vi "Teleop.vi"(10 "Match Info":T7={"Autonomous Elapsed Seconds"=0.0, "TeleOp Elapsed Seconds"=0.0, "Disabled Elapsed Seconds"=0.0, "Visited Autonomous"=FALSE, "Visited TeleOp"=FALSE, "Visited Disabled"=FALSE, "Autonomous Settings"={"Autonomous Style"=enum."Independent", "VI Refnum"=refnum}}, 11 "Call Context":T8) -> ()   [LabVIEW 2013]
doc: "This VI is called for each TeleOp packet received from the DS where the robot is not disabled. It is often used to read from the joysticks and update I/O or to update setpoints for timed control loops. It should complete and return within 20 milliseconds or it may miss DS packets."
uses:
  <vilib>/Rock Robotics/WPI/DriverStation/WPI_DriverStationDerivedRobotMode.ctl
  <vilib>/Rock Robotics/WPI/DriverStation/WPI_DriverStationMatch Info.ctl
  <vilib>/Rock Robotics/WPI/Joystick/WPI_JoystickButtonState.ctl
  <vilib>/Rock Robotics/WPI/Relay/WPI_RelayDevRef.ctl
  <vilib>/Rock Robotics/SystemInterfaces/DIO/FPGA_DIORelayChannel.ctl
  <vilib>/Rock Robotics/SystemInterfaces/Typedef/FPGA_TypedefDigitalModule.ctl
  <vilib>/Rock Robotics/WPI/Relay/WPI_RelayDirection.ctl
  <vilib>/Rock Robotics/WPI/DriverStation/DriverStationLCD/WPI_DriverStationLCDLCDLine.ctl
  <vilib>/Rock Robotics/WPI/Relay/WPI_RelayValue.ctl
  Robot Global Data.vi
  <vilib>/addons/control/pid/pid.llb/PID (DBL).vi
  <vilib>/Rock Robotics/WPI/RobotDrive/WPI_RobotDriveArcadeDrive_Standard(NoSaturation).vi
  <vilib>/Rock Robotics/WPI/RobotDrive/WPI_RobotDriveGetSetRefNum.vi
  <vilib>/Rock Robotics/WPI/Joystick/WPI_JoystickGetSetRefNum.vi
  <vilib>/addons/control/pid/NI_PID_pid.lvlib
panel:
  out "trimmert_watch":i32
  in  "steering_trim":dbl(slide) scale=1.0..-1.0
  in  "Ball_Sucker_Reducer":dbl=0.8
  in  "shooter_speed_med_high":dbl(slide)=0.6 scale=0.0..1.0
  in  "shooter_speed_med_low":dbl(slide)=0.35 scale=0.0..1.0
  in  "shooter_speed_high":dbl(slide)=1.0 scale=0.0..1.0
  in  "shooter_speed_low":dbl(slide)=0.25 scale=0.0..1.0
  in  "Camera_Tilt_Position":dbl(slide)=0.55 scale=1.0..-1.0
  in  "Shoot_Feeder_Reducer":dbl=0.9
  out "Battery_Relay":T1={"DevStatus"={"status"=FALSE, "code"=0, "source"=""}, "Relay Channel"=enum."Invalid", "Digital Module"=enum."Digital Module 1", "Relay Direction"=enum."Both directions"}
  in  "Camera_Pan_Position":dbl(slide)=-1.0 scale=1.0..-1.0
  in  "ARM_HOME":dbl(slide)=0.53 scale=1.0..-1.0
  in  "ARM_REV_LIMIT":dbl(slide)=-0.2 scale=1.0..-1.0
  in  "Drive_Y_Speed":dbl
  in  "Drive_X_Speed":dbl=1.5
  in  "Feeder_Arm_Speed":dbl
  in  "Sucker_Speed":dbl
  in  "Shooter_Speed":dbl=1.5
  in  "Shoot_Feeder_Speed":dbl=1.5
  in  "Ball_Sucker_Threshold":i64=10
  in  "Ball_Sucker_Delay_ms":i64=100
  in  "Ball_Sucker_Counter":i64
  in  "Steering_Reduce":dbl=2.0
  in  "Shooter_Angle_Raw":dbl
  in  "Camera_SIDE_Val":dbl=0.5
  in  "Camera_FWD_Val":dbl
  in  "ARM_FWD_LIMIT":dbl(slide)=0.53 scale=1.0..-1.0
  in  "Drive_Reduce":dbl=0.75
  out "JS1_BTNS":T5
  out "JS1_AXES":T6
  out "JS2_BTNS":T5
  out "JS2_AXES":T6
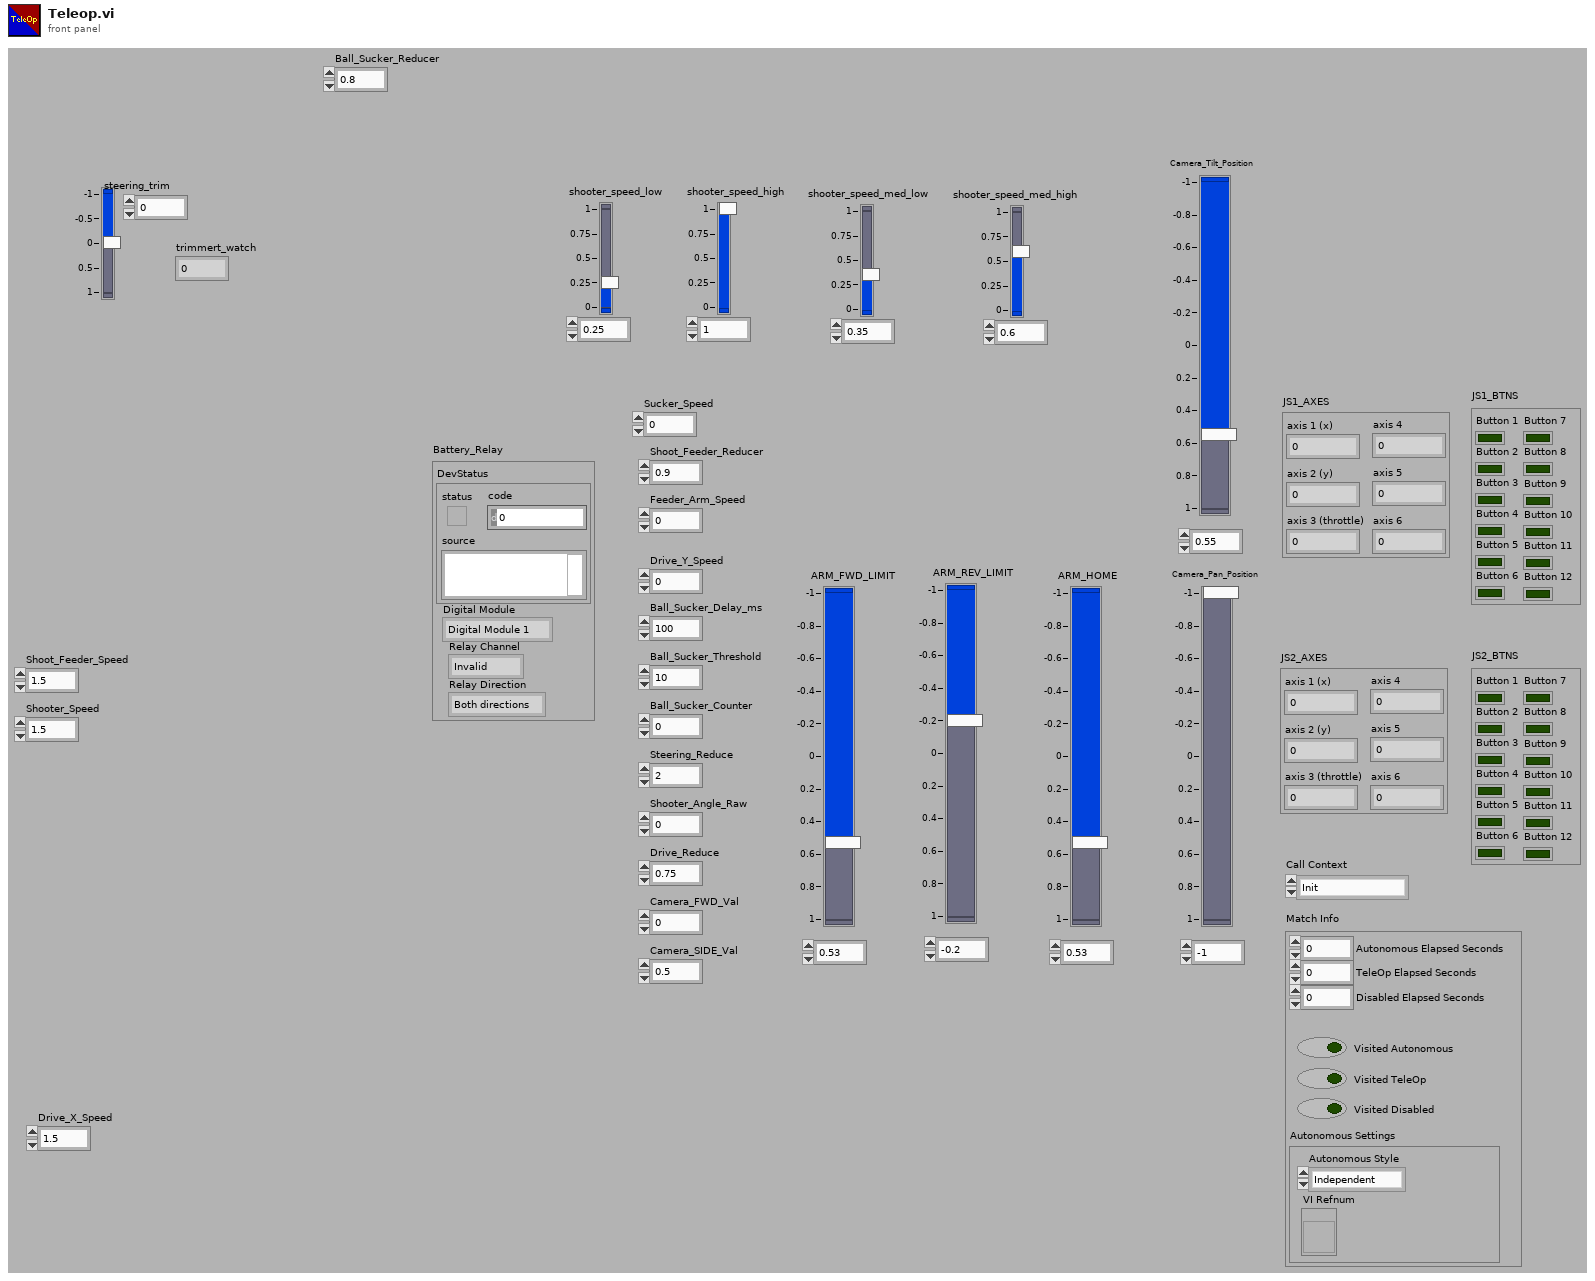
[diagram p1: front panel]
types:
  T1 = typedef "WPI_RelayDevRef.ctl" = cluster{"DevStatus":errorcluster, "Relay Channel":T2, "Digital Module":T3, "Relay Direction":T4}
  T2 = typedef "FPGA_DIORelayChannel.ctl" = enum8{"Relay 1", "Relay 2", "Relay 3", "Relay 4", "Relay 5", "Relay 6", "Relay 7", "Relay 8", "Invalid"}
  T3 = typedef "FPGA_TypedefDigitalModule.ctl" = enum16{"Digital Module 1", "Digital Module 2"}
  T4 = typedef "WPI_RelayDirection.ctl" = enum16{"Both directions", "Forward only", "Reverse only"}
  T5 = typedef "WPI_JoystickButtonState.ctl" = cluster{"Button 1":bool, "Button 2":bool, "Button 3":bool, "Button 4":bool, "Button 5":bool, "Button 6":bool, "Button 7":bool, "Button 8":bool, "Button 9":bool, "Button 10":bool, "Button 11":bool, "Button 12":bool}
  T6 = cluster{"axis 1 (x)":dbl, "axis 2 (y)":dbl, "axis 3 (throttle)":dbl, "axis 4":dbl, "axis 5":dbl, "axis 6":dbl}
  T7 = typedef "WPI_DriverStationMatch Info.ctl" = cluster{"Autonomous Elapsed Seconds":dbl, "TeleOp Elapsed Seconds":dbl, "Disabled Elapsed Seconds":dbl, "Visited Autonomous":bool, "Visited TeleOp":bool, "Visited Disabled":bool, "Autonomous Settings":cluster{"Autonomous Style":enum16{"Iterative", "Independent"}, "VI Refnum":refnum<vi>}}
  T8 = typedef "WPI_DriverStationDerivedRobotMode.ctl" = enum16{"Init", "Execute", "Stop"}
  T9 = typedef "WPI_DriverStationLCDLCDLine.ctl" = enum16{"Main - Line 1", "User - Line 2", "User - Line 3", "User - Line 4", "User - Line 5", "User - Line 6"}
  T10 = typedef "WPI_JoystickDevRef.ctl" = cluster{"Device":T11}
  T11 = typedef "WPI_JoystickDeviceEnum.ctl" = enum16{"USB 1", "USB 2", "USB 3", "USB 4", "Kinect 1", "Kinect 2"}
  T12 = typedef "WPI_MotorControlDeviceRef.ctl" = cluster{"DeviceStatus":errorcluster, "Type":enum16{"PWM", "CAN"}, "PWM":cluster{"Digital Module":T3, "PWM Channel":T13, "DeadBand":T14}, "CAN":cluster{"Device Number":u8, "Control Mode":T15, "Semaphore":T16, "Max Vout":dbl}, "Invert":bool, "TransformRef":T17, "InvTransformRef":T17}
  T13 = typedef "FPGA_DIOPWMChannel.ctl" = enum8{"PWM 1", "PWM 2", "PWM 3", "PWM 4", "PWM 5", "PWM 6", "PWM 7", "PWM 8", "PWM 9", "PWM 10", "Invalid"}
  T14 = typedef "WPI_PWMDeadband.ctl" = cluster{"Name":string, "maxPositivePwm":i32, "minPositivePwm":i32, "centerPwm":i32, "maxNegativePwm":i32, "minNegativePwm":i32, "angularRange":u16}
  T15 = typedef "WPI_CANJaguar_ControlMode.ctl" = enum8{"Percent VBus", "Current", "Speed", "Position", "Voltage"}
  T16 = typedef "Semaphore RefNum" = refnum<k1>
  T17 = typedef "WPI_PWMTransform_ConPane.ctl" = refnum<vi>
  T18 = typedef "WPI_RobotDriveDevRef.ctl" = cluster{"DevStatus":errorcluster, "Motors[]":T12[], "Square Inputs":bool, "Max Output":dbl, "Isochronous":bool}
  T19 = cluster{"proportional gain (Kc)":dbl, "integral time (Ti, min)":dbl, "derivative time (Td, min)":dbl}
  T20 = typedef "WPI_AnalogChannelDevRef.ctl" = cluster{"DevStatus":errorcluster, "Analog Module":T21, "Analog Channel":T22}
  T21 = typedef "FPGA_TypedefAnalogModule.ctl" = enum16{"Analog Module 1", "Analog Module 2"}
  T22 = typedef "FPGA_AIChannel.ctl" = enum8{"AI 1", "AI 2", "AI 3", "AI 4", "AI 5", "AI 6", "AI 7", "AI 8", "Invalid"}
  T23 = typedef "WPI_RelayValue.ctl" = enum16{"Off", "On", "Forward", "Reverse"}
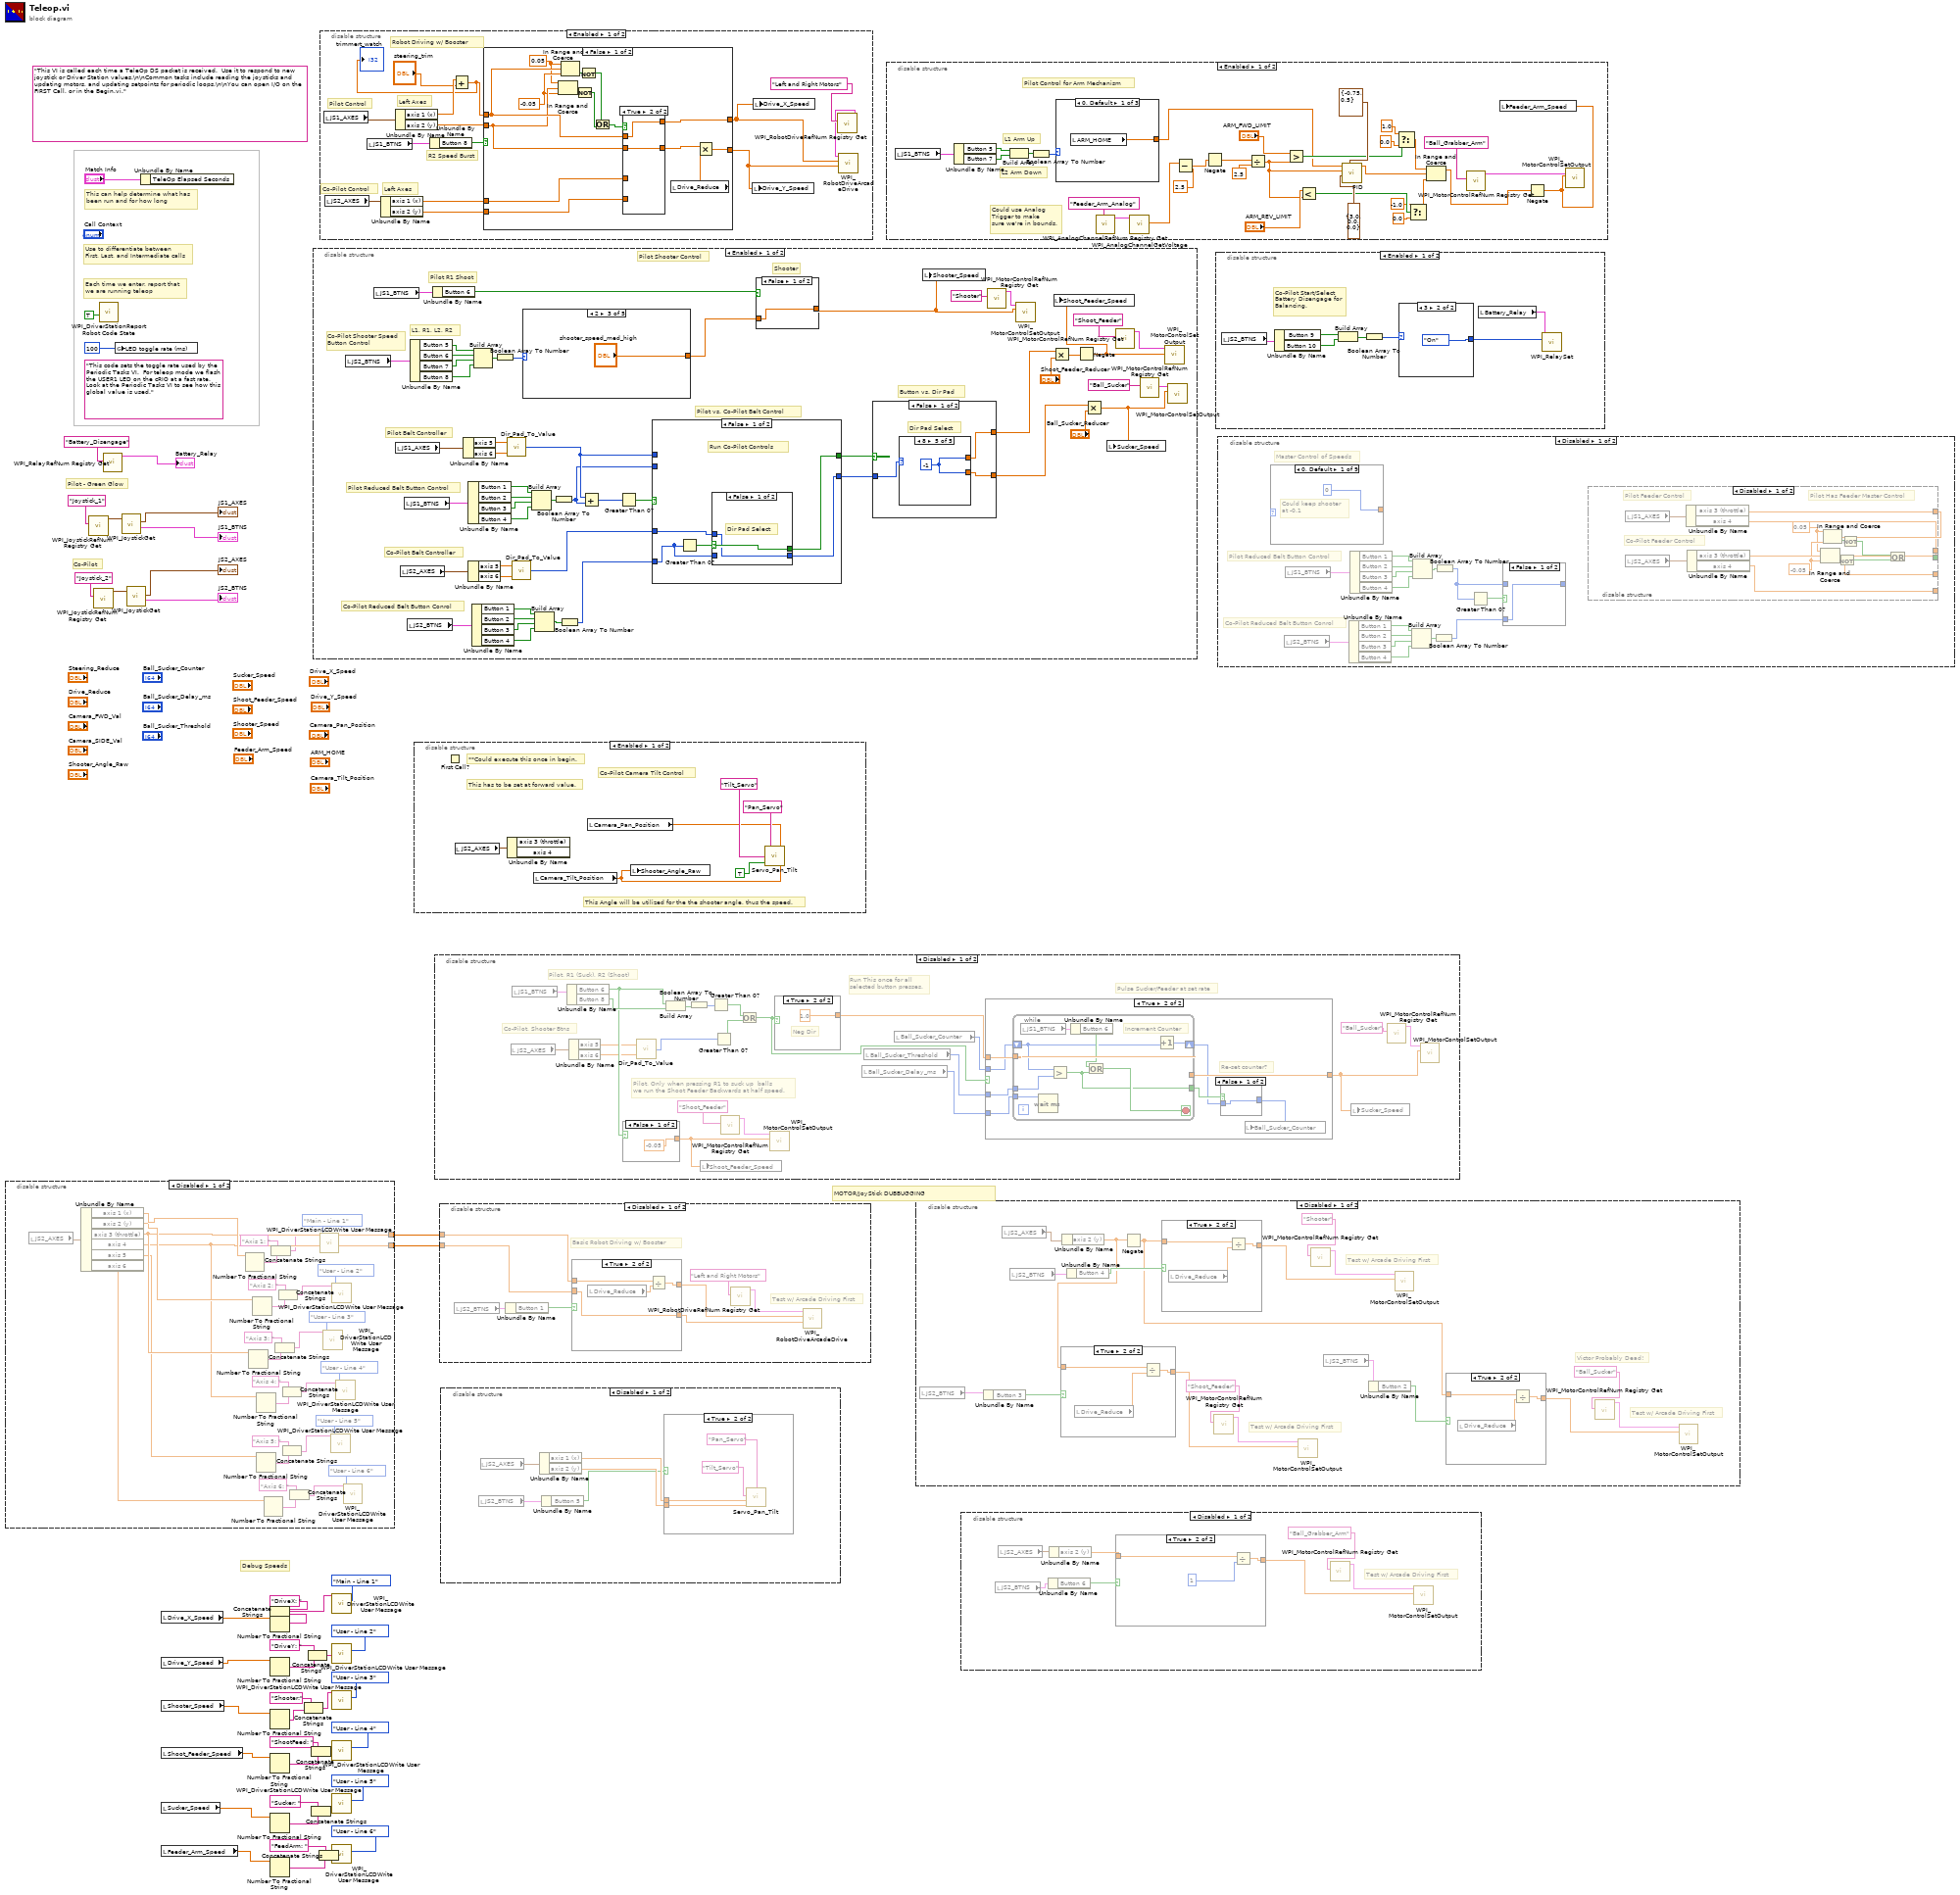
[diagram p0: block diagram]
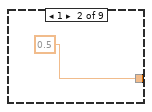
[diagram p4: hidden frame]
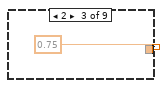
[diagram p5: hidden frame]
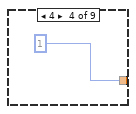
[diagram p6: hidden frame]
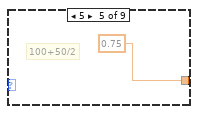
[diagram p7: hidden frame]
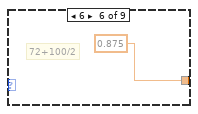
[diagram p8: hidden frame]
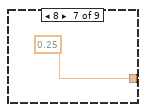
[diagram p9: hidden frame]
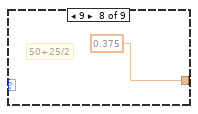
[diagram p10: hidden frame]
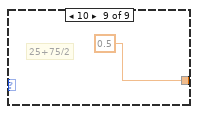
[diagram p11: hidden frame]
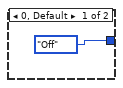
[diagram p13: hidden frame]
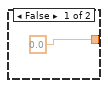
[diagram p16: hidden frame]
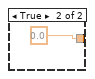
[diagram p18: hidden frame]
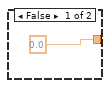
[diagram p19: hidden frame]
diagram:
  (unwired) "This code sets the toggle rate used by the Periodic Tasks VI.  For teleop mode we flash the USER1 LED on the cRIO at a fast rate.  Look at the Periodic Tasks VI to see how this global value is used."
  (unwired) "This VI is called each time a TeleOp DS packet is received.  Use it to respond to new joystick or Driver Station values.\n\nCommon tasks include reading the joysticks and updating motors, and updating setpoints for periodic loops.\n\nYou can open I/O on the FIRST Call, or in the Begin.vi."
  # "Debug Speeds"
  # "Co-Pilot"
  # "Pilot - Green Glow"
  # "MOTOR/JoyStick DUBBUGGING"
  # "Each time we enter, report that\nwe are running teleop"
  # "Use to differentiate between\nFirst, Last, and Intermediate calls"
  # "This can help determine what has\nbeen run and for how long"
  n1 = disable-structure shown="Disabled" {
    disable-tunnel: [w73 _] -> w34
    disable-tunnel: [w72 _] -> w33
    frame Disabled {
      n2 = local read "JS2_AXES"() -> (w76:T6)
      n3 = Unbundle By Name(w76) -> ("axis 1 (x)"=w75:dbl, "axis 2 (y)"=w74:dbl, "axis 3 (throttle)"=w73:dbl, "axis 4"=w72:dbl, "axis 5"=w71:dbl, "axis 6"=w70:dbl)
      n4 = Number To Fractional String(number=w75) -> (F-format string=w67:string)  [unwired: 3 in]
      n5 = Number To Fractional String(number=w73) -> (F-format string=w59:string)  [unwired: 3 in]
      n6 = Number To Fractional String(number=w74) -> (F-format string=w65:string)  [unwired: 3 in]
      n7 = Number To Fractional String(number=w72) -> (F-format string=w57:string)  [unwired: 3 in]
      n8 = Number To Fractional String(number=w71) -> (F-format string=w51:string)  [unwired: 3 in]
      n9 = Number To Fractional String(number=w70) -> (F-format string=w49:string)  [unwired: 3 in]
      n10 = Concatenate Strings("Axis 1: ", w67) -> (w64:string)
      n11 = Concatenate Strings("Axis 3: ", w59) -> (w56:string)
      n12 = Concatenate Strings("Axis 2: ", w65) -> (w62:string)
      n13 = Concatenate Strings("Axis 4: ", w57) -> (w54:string)
      n14 = Concatenate Strings("Axis 5: ", w51) -> (w48:string)
      n15 = Concatenate Strings("Axis 6: ", w49) -> (w46:string)
      n16 = call <vilib>:"WPI_DriverStationLCDWrite User Message.vi"("line text"=w64, "line"=WPI_DriverStationLCDLCDLine."Main - Line 1") -> ()  [unwired: 13 in, 1 out]
      n17 = call <vilib>:"WPI_DriverStationLCDWrite User Message.vi"("line text"=w56, "line"=WPI_DriverStationLCDLCDLine."User - Line 3") -> ()  [unwired: 13 in, 1 out]
      n18 = call <vilib>:"WPI_DriverStationLCDWrite User Message.vi"("line text"=w48, "line"=WPI_DriverStationLCDLCDLine."User - Line 5") -> ()  [unwired: 13 in, 1 out]
      n19 = call <vilib>:"WPI_DriverStationLCDWrite User Message.vi"("line text"=w62, "line"=WPI_DriverStationLCDLCDLine."User - Line 2") -> ()  [unwired: 13 in, 1 out]
      n20 = call <vilib>:"WPI_DriverStationLCDWrite User Message.vi"("line text"=w54, "line"=WPI_DriverStationLCDLCDLine."User - Line 4") -> ()  [unwired: 13 in, 1 out]
      n21 = call <vilib>:"WPI_DriverStationLCDWrite User Message.vi"("line text"=w46, "line"=WPI_DriverStationLCDLCDLine."User - Line 6") -> ()  [unwired: 13 in, 1 out]
    }
    frame Enabled {
    }
  }
  n22 = call <vilib>:"WPI_JoystickRefNum Registry Get.vi"("refnum name"="Joystick_1") -> ("JoystickDevRef"=w38:T10)  [unwired: 1 in, 9 out]
  n23 = call <vilib>:"WPI_JoystickRefNum Registry Get.vi"("refnum name"="Joystick_2") -> ("JoystickDevRef"=w40:T10)  [unwired: 1 in, 9 out]
  n24 = call <vilib>:"WPI_DriverStationReport Robot Code State.vi"("TeleOp"=TRUE ("Autonomous")) -> ()  [unwired: 10 in, 1 out]
  n25 = call <vilib>:"WPI_RelayRefNum Registry Get.vi"("refnum name"="Battery_Disengage") -> ("RelayDevRef"=→"Battery_Relay":T1)  [unwired: 9 in, 1 out]
  n26 = global write "Robot Global Data.vi" "LED toggle rate (ms)"(u32 100 ("LED ms toggle rate")) -> ()
  n27 = call <vilib>:"WPI_JoystickGet.vi"("JoystickDevRef"=w38) -> ("Buttons"=→"JS1_BTNS":T5, "Axes"=→"JS1_AXES":T6)  [unwired: 1 in, 4 out]
  n28 = call <vilib>:"WPI_JoystickGet.vi"("JoystickDevRef"=w40) -> ("Buttons"=→"JS2_BTNS":T5, "Axes"=→"JS2_AXES":T6)  [unwired: 1 in, 4 out]
  n29 = Unbundle By Name("Match Info") -> ()  [unwired: 1 out]
  n30 = local read "Drive_X_Speed"() -> (w9:dbl)
  n31 = local read "Drive_Y_Speed"() -> (w8:dbl)
  n32 = local read "Shooter_Speed"() -> (w7:dbl)
  n33 = local read "Shoot_Feeder_Speed"() -> (w6:dbl)
  n34 = local read "Sucker_Speed"() -> (w5:dbl)
  n35 = local read "Feeder_Arm_Speed"() -> (w4:dbl)
  n36 = Number To Fractional String(number=w9) -> (F-format string=w30:string)  [unwired: 3 in]
  n37 = Concatenate Strings("DriveX: ", w30) -> (w27:string)
  n38 = Number To Fractional String(number=w8) -> (F-format string=w28:string)  [unwired: 3 in]
  n39 = Number To Fractional String(number=w7) -> (F-format string=w3:string)  [unwired: 3 in]
  n40 = Number To Fractional String(number=w6) -> (F-format string=w21:string)  [unwired: 3 in]
  n41 = Number To Fractional String(number=w5) -> (F-format string=w15:string)  [unwired: 3 in]
  n42 = Number To Fractional String(number=w4) -> (F-format string=w13:string)  [unwired: 3 in]
  n43 = Concatenate Strings("Shooter:", w3) -> (w20:string)
  n44 = Concatenate Strings("DriveY: ", w28) -> (w25:string)
  n45 = Concatenate Strings("ShootFeed: ", w21) -> (w18:string)
  n46 = Concatenate Strings("Sucker: ", w15) -> (w12:string)
  n47 = disable-structure shown="Enabled" {
    frame Enabled {
      # "Button vs. Dir Pad"
      # "Pilot vs. Co-Pilot Belt Control"
      # "Co-Pilot Belt Controller"
      # "L1, R1, L2, R2"
      # "Co-Pilot Reduced Belt Button Conrol"
      # "Pilot Reduced Belt Button Control"
      # "Pilot Belt Controller"
      # "Co-Pilot Shooter Speed\nButton Control"
      # "Pilot R1 Shoot"
      # "Shooter"
      # "Pilot Shooter Control"
      n48 = local read "JS2_BTNS"() -> (w108:T5)
      n49 = local read "JS1_BTNS"() -> (w126:T5)
      n50 = local read "JS1_AXES"() -> (w105:T6)
      n51 = local read "JS2_AXES"() -> (w90:T6)
      n52 = local read "JS1_BTNS"() -> (w104:T5)
      n53 = local read "JS2_BTNS"() -> (w93:T5)
      n54 = Unbundle By Name(w108) -> ("Button 5"=w114:bool, "Button 6"=w113:bool, "Button 7"=w112:bool, "Button 8"=w111:bool)
      n55 = Unbundle By Name(w126) -> ("Button 6"=w117:bool)
      n56 = Unbundle By Name(w105) -> ("axis 5"=w107:dbl, "axis 6"=w106:dbl)
      n57 = Unbundle By Name(w104) -> ("Button 1"=w99:bool, "Button 2"=w100:bool, "Button 3"=w101:bool, "Button 4"=w102:bool)
      n58 = Unbundle By Name(w90) -> ("axis 5"=w88:dbl, "axis 6"=w89:dbl)
      n59 = Unbundle By Name(w93) -> ("Button 1"=w98:bool, "Button 2"=w97:bool, "Button 3"=w96:bool, "Button 4"=w95:bool)
      n60 = Build Array(w114, w113, w112, w111) -> (w110:bool[])
      n61 = Boolean Array To Number(Boolean array=w110) -> (number=w109:u32)
      n62 = call "Dir_Pad_To_Value.vi"("Axis_6_Val"=w106, "Axis_5_Val"=w107) -> ("Pos_Pad_Val"=w84:i32)
      n63 = call "Dir_Pad_To_Value.vi"("Axis_6_Val"=w89, "Axis_5_Val"=w88) -> ("Pos_Pad_Val"=w82:i32)
      n64 = case shown="2" w109 {
        tunnel: [0 "shooter_speed_med_low" "shooter_speed_med_high" "shooter_speed_low" "shooter_speed_high"] -> w91
        frame 0, Default {
          # "Keep shooter\non so its easy\nto get up to \nspeed?"
        }
        frame 1 {
        }
        frame 2 {
        }
        frame 4 {
        }
        frame 8 {
        }
      }
      n65 = Build Array(w99, w100, w101, w102) -> (w103:bool[])
      n66 = Build Array(w98, w97, w96, w95) -> (w94:bool[])
      n67 = Boolean Array To Number(Boolean array=w103) -> (number=w83:u32)
      n68 = Boolean Array To Number(Boolean array=w94) -> (number=w81:u32)
      n69 = Add(x=w84, y=w83) -> (x+y=w86:u32)
      n70 = Greater Than 0?(x=w86) -> (x > 0?=w85:bool)
      n71 = case shown="False" w85 {
        tunnel: w84 -> [_ w162]
        tunnel: w83 -> [_ w161]
        tunnel: w82 -> [w153 _]
        tunnel: w81 -> [w150 _]
        tunnel: [w152 w160] -> w80
        tunnel: [w151 w159] -> w77
        frame False {
          # "Run Co-Pilot Controls"
          n72 = Greater Than 0?(x=w150) -> (x > 0?=w154:bool)
          n73 = case shown="False" w154 {
            selector: w154 -> [w156 w158]
            tunnel: w153 -> [w155 _]
            tunnel: [w155 w157] -> w151
            tunnel: [w156 w158] -> w152
            tunnel: w150 -> [_ w157]
            frame False {
              # "Dir Pad Select"
            }
            frame True {
              # "Button Select"
            }
          }
        }
        frame True {
          # "Run Pilot Controls"
          n74 = Greater Than 0?(x=w161) -> (x > 0?=w163:bool)
          n75 = case shown="False" w163 {
            selector: w163 -> [w164 w166]
            tunnel: w162 -> [w165 _]
            tunnel: w161 -> [_ w167]
            tunnel: [w165 w167] -> w159
            tunnel: [w164 w166] -> w160
            frame False {
              # "Dir Pad Select"
            }
            frame True {
              # "Button Select"
            }
          }
        }
      }
      n76 = case shown="False" w117 {
        tunnel: w91 -> [w173 _]
        tunnel: [w173 1.0] -> w118
        frame False {
        }
        frame True {
        }
      }
      n77 = case shown="False" w80 {
        tunnel: [w129 w140] -> w79
        tunnel: [w128 w139] -> w78
        tunnel: w77 -> [w127 w138]
        frame False {
          # "Dir Pad Select"
          n78 = case shown="8" w127 {
            tunnel: [w130 1 -1.0 1 w137] -> w128
            tunnel: [w130 -1 1 1.0 w137] -> w129
            frame 0, Default {
              w130 = 0.0
            }
            frame 1 {
            }
            frame 2 {
            }
            frame 4 {
            }
            frame 8 {
              w137 = -1
            }
          }
        }
        frame True {
          # "Button Select"
          n79 = case shown="8" w138 {
            tunnel: [w141 -1 0 1 0] -> w139
            tunnel: [w141 0 -1.0 0 1.0] -> w140
            frame 0, Default {
              w141 = 0.0
            }
            frame 1 {
            }
            frame 2 {
            }
            frame 4 {
            }
            frame 8 {
            }
          }
        }
      }
      n80 = local write "Shooter_Speed"(w118) -> ()
      n81 = call <vilib>:"WPI_MotorControlRefNum Registry Get.vi"("refnum name"="Shooter") -> ("MotorControlDevRef"=w124:T12)  [unwired: 9 in, 1 out]
      n82 = call <vilib>:"WPI_MotorControlSetOutput.vi"("Output"=w118, "MotorControlDevRef"=w124) -> ()  [unwired: 7 in, 3 out]
      n83 = Multiply(x=w79, y="Shoot_Feeder_Reducer") -> (x*y=w116:dbl)
      n84 = Negate(x=w116) -> (-x=w121:dbl)
      n85 = local write "Shoot_Feeder_Speed"(w121) -> ()
      n86 = Multiply(x=w78, y="Ball_Sucker_Reducer") -> (x*y=w87:dbl)
      n87 = local write "Sucker_Speed"(w87) -> ()
      n88 = call <vilib>:"WPI_MotorControlRefNum Registry Get.vi"("refnum name"="Shoot_Feeder") -> ("MotorControlDevRef"=w122:T12)  [unwired: 9 in, 1 out]
      n89 = call <vilib>:"WPI_MotorControlRefNum Registry Get.vi"("refnum name"="Ball_Sucker") -> ("MotorControlDevRef"=w119:T12)  [unwired: 9 in, 1 out]
      n90 = call <vilib>:"WPI_MotorControlSetOutput.vi"("Output"=w121, "MotorControlDevRef"=w122) -> ()  [unwired: 7 in, 3 out]
      n91 = call <vilib>:"WPI_MotorControlSetOutput.vi"("Output"=w87, "MotorControlDevRef"=w119) -> ()  [unwired: 7 in, 3 out]
    }
    frame Disabled {
    }
  }
  n92 = Concatenate Strings("FeedArm: ", w13) -> (w10:string)
  n93 = disable-structure shown="Enabled" {
    frame Enabled {
      # "Left Axes"
      # "Left Axes"
      # "Co-Pilot Control"
      # "Pilot Control"
      # "R2 Speed Burst"
      # "Robot Driving w/ Booster"
      n94 = local read "JS1_AXES"() -> (w186:T6)
      n95 = local read "JS2_AXES"() -> (w181:T6)
      n96 = local read "JS1_BTNS"() -> (w185:T5)
      n97 = Unbundle By Name(w181) -> ("axis 1 (x)"=w180:dbl, "axis 2 (y)"=w179:dbl)
      n98 = Unbundle By Name(w186) -> ("axis 1 (x)"=w177:dbl, "axis 2 (y)"=w184:dbl)
      n99 = Unbundle By Name(w185) -> ("Button 8"=w183:bool)
      n100 = Add(x=w177, y="steering_trim") -> (x+y=w175:dbl)
      "trimmert_watch" <- w175
      n101 = case shown="False" w183 {
        tunnel: w184 -> [w194 w208]
        tunnel: [w202 w208] -> w182
        tunnel: w175 -> [w195 w209]
        tunnel: [w199 w209] -> w178
        tunnel: w180 -> [w201 _]
        tunnel: w179 -> [w198 _]
        frame False {
          w190 = -0.05
          w189 = 0.05
          n102 = In Range and Coerce(upper limit=w189, x=w194, lower limit=w190) -> (In Range?=w196:bool)  [unwired: 1 out]
          n103 = In Range and Coerce(upper limit=w189, x=w195, lower limit=w190) -> (In Range?=w197:bool)  [unwired: 1 out]
          n104 = Not(x=w196) -> (.not. x?=w192:bool)
          n105 = Not(x=w197) -> (.not. x?=w193:bool)
          n106 = Or(x=w193, y=w192) -> (x .or. y?=w191:bool)
          n107 = case shown="True" w191 {
            tunnel: w201 -> [w205 _]
            tunnel: [w204 w207] -> w200
            tunnel: [w205 w206] -> w199
            tunnel: w195 -> [_ w206]
            tunnel: w194 -> [_ w207]
            tunnel: w198 -> [w204 _]
            frame False {
            }
            frame True {
            }
          }
          n108 = local read "Drive_Reduce"() -> (w203:dbl)
          n109 = Multiply(x=w200, y=w203) -> (x*y=w202:dbl)
        }
        frame True {
        }
      }
      n110 = local write "Drive_Y_Speed"(w182) -> ()
      n111 = local write "Drive_X_Speed"(w178) -> ()
      n112 = call <vilib>:"WPI_RobotDriveRefNum Registry Get.vi"("refnum name"="Left and Right Motors") -> ("RobotDriveDevRef"=w187:T18)  [unwired: 1 in, 9 out]
      n113 = call-poly <vilib>:"WPI_RobotDriveArcadeDrive.vi"("Y axis value"=w182, "X axis value"=w178, "RobotDriveDevRef"=w187) -> ()  [unwired: 6 in, 3 out]
    }
    frame Disabled {
    }
  }
  n114 = call <vilib>:"WPI_DriverStationLCDWrite User Message.vi"("line text"=w27, "line"=WPI_DriverStationLCDLCDLine."Main - Line 1") -> ()  [unwired: 13 in, 1 out]
  n115 = call <vilib>:"WPI_DriverStationLCDWrite User Message.vi"("line text"=w25, "line"=WPI_DriverStationLCDLCDLine."User - Line 2") -> ()  [unwired: 13 in, 1 out]
  n116 = call <vilib>:"WPI_DriverStationLCDWrite User Message.vi"("line text"=w20, "line"=WPI_DriverStationLCDLCDLine."User - Line 3") -> ()  [unwired: 13 in, 1 out]
  n117 = call <vilib>:"WPI_DriverStationLCDWrite User Message.vi"("line text"=w18, "line"=WPI_DriverStationLCDLCDLine."User - Line 4") -> ()  [unwired: 13 in, 1 out]
  n118 = call <vilib>:"WPI_DriverStationLCDWrite User Message.vi"("line text"=w12, "line"=WPI_DriverStationLCDLCDLine."User - Line 5") -> ()  [unwired: 13 in, 1 out]
  n119 = call <vilib>:"WPI_DriverStationLCDWrite User Message.vi"("line text"=w10, "line"=WPI_DriverStationLCDLCDLine."User - Line 6") -> ()  [unwired: 13 in, 1 out]
  n120 = disable-structure shown="Enabled" {
    frame Enabled {
      # "**Could execute this once in begin."
      # "This Angle will be utilized for the the shooter angle, thus the speed."
      # "This has to be set at forward value."
      # "Co-Pilot Camera Tilt Control"
      n121 = First Call?() -> ()  [unwired: 1 out]
      n122 = local read "JS2_AXES"() -> (w215:T6)
      n123 = Unbundle By Name(w215) -> ()  [unwired: 2 out]
      n124 = local read "Camera_Tilt_Position"() -> (w210:dbl)
      n125 = local read "Camera_Pan_Position"() -> (w211:dbl)
      n126 = local write "Shooter_Angle_Raw"(w210) -> ()
      n127 = call "Servo_Pan_Tilt.vi"("Tilt_Servo_Position"=w210, "Pan_Servo_Position"=w211, "Smooth?"=TRUE, "Tilt_Servo_Name"="Tilt_Servo", "Pan_Servo_Name"="Pan_Servo") -> ()
    }
    frame Disabled {
    }
  }
  n128 = disable-structure shown="Disabled" {
    frame Disabled {
      # "Pilot, Only when pressing R1 to suck up  balls\nwe run the Shoot Feeder Backwards at half speed."
      # "Co-Pilot, Shooter Btns"
      # "Pilot, R1 (Suck), R2 (Shoot)"
      # "Run This once for all\nselected button presses."
      # "Pulse Sucker/Feeder at set rate"
      n129 = local read "JS2_AXES"() -> (w221:T6)
      n130 = local read "JS1_BTNS"() -> (w231:T5)
      n131 = Unbundle By Name(w231) -> ("Button 6"=w222:bool, "Button 8"=w230:bool)
      n132 = Unbundle By Name(w221) -> ("axis 5"=w219:dbl, "axis 6"=w220:dbl)
      n133 = case shown="False" w222 {
        tunnel: [-0.05 0.0] -> w216
        frame False {
        }
        frame True {
        }
      }
      n134 = call "Dir_Pad_To_Value.vi"("Axis_6_Val"=w220, "Axis_5_Val"=w219) -> ("Pos_Pad_Val"=w218:i32)
      n135 = Build Array(w222, w230) -> (w229:bool[])
      n136 = Boolean Array To Number(Boolean array=w229) -> (number=w228:u32)
      n137 = local write "Shoot_Feeder_Speed"(w216) -> ()
      n138 = Greater Than 0?(x=w228) -> (x > 0?=w226:bool)
      n139 = Greater Than 0?(x=w218) -> (x > 0?=w225:bool)
      n140 = call <vilib>:"WPI_MotorControlRefNum Registry Get.vi"("refnum name"="Shoot_Feeder") -> ("MotorControlDevRef"=w223:T12)  [unwired: 9 in, 1 out]
      n141 = Or(x=w226, y=w225) -> (x .or. y?=w227:bool)
      n142 = call <vilib>:"WPI_MotorControlSetOutput.vi"("Output"=w216, "MotorControlDevRef"=w223) -> ()  [unwired: 7 in, 3 out]
      n143 = case shown="True" w227 {
        tunnel: [0.0 1.0] -> w232
        frame False {
        }
        frame True {
          # "Neg Dir"
        }
      }
      n144 = local read "Ball_Sucker_Delay_ms"() -> (w234:i64)
      n145 = local read "Ball_Sucker_Threshold"() -> (w233:i64)
      n146 = local read "Ball_Sucker_Counter"() -> (w235:i64)
      n147 = case shown="True" w227 {
        tunnel: [w242 w247] -> w217
        tunnel: w232 -> [w242 w248]
        tunnel: w235 -> [_ w246]
        tunnel: w234 -> [_ w250]
        tunnel: w233 -> [_ w249]
        frame False {
          # "Do not update counter value."
        }
        frame True {
          # "Re-set counter?"
          n148 = while {
            tunnel: [w257] -> w247
            tunnel: w250 -> [w261]
            tunnel: w249 -> [w259]
            tunnel: w248 -> [w257]
            shift-right: [w255] -> w244
            shift-left: w246 -> [w254]
            tunnel: [w253] -> w245
            stop <- w260 stop-if-true
            # "Increment Counter"
            n149 = local read "JS1_BTNS"() -> (w258:T5)
            n150 = Wait (ms)(milliseconds to wait=w261) -> ()  [unwired: 1 out]
            n151 = Greater?(x=w254, y=w259) -> (0:w253:bool)
            n152 = Unbundle By Name(w258) -> ("Button 6"=w256:bool)
            n153 = Or(x=w256, y=w253) -> (x .or. y?=w260:bool)
            n154 = Increment(x=w254) -> (x+1=w255:i64)
          }
          n155 = case shown="False" w245 {
            tunnel: w244 -> [w251 _]
            tunnel: [w251 0] -> w243
            frame False {
            }
            frame True {
            }
          }
          n156 = local write "Ball_Sucker_Counter"(w243) -> ()
        }
      }
      n157 = local write "Sucker_Speed"(w217) -> ()
      n158 = call <vilib>:"WPI_MotorControlRefNum Registry Get.vi"("refnum name"="Ball_Sucker") -> ("MotorControlDevRef"=w236:T12)  [unwired: 9 in, 1 out]
      n159 = call <vilib>:"WPI_MotorControlSetOutput.vi"("Output"=w217, "MotorControlDevRef"=w236) -> ()  [unwired: 7 in, 3 out]
    }
    frame Enabled {
    }
  }
  n160 = disable-structure shown="Disabled" {
    disable-tunnel: w34 -> [w263 _]
    disable-tunnel: w33 -> [w262 _]
    frame Disabled {
      # "Basic Robot Driving w/ Booster"
      # "Test w/ Arcade Driving First"
      n161 = local read "JS2_BTNS"() -> (w267:T5)
      n162 = Unbundle By Name(w267) -> ("Button 1"=w264:bool)
      n163 = case shown="True" w264 {
        tunnel: w262 -> [_ w272]
        tunnel: [w270 w272] -> w265
        tunnel: w263 -> [_ w274]
        tunnel: [w270 w273] -> w266
        frame False {
          w270 = 0.0
        }
        frame True {
          n164 = local read "Drive_Reduce"() -> (w271:dbl)
          n165 = Divide(x=w274, y=w271) -> (x/y=w273:dbl)
        }
      }
      n166 = call <vilib>:"WPI_RobotDriveRefNum Registry Get.vi"("refnum name"="Left and Right Motors") -> ("RobotDriveDevRef"=w268:T18)  [unwired: 1 in, 9 out]
      n167 = call-poly <vilib>:"WPI_RobotDriveArcadeDrive.vi"("Y axis value"=w265, "X axis value"=w266, "RobotDriveDevRef"=w268) -> ()  [unwired: 6 in, 3 out]
    }
    frame Enabled {
    }
  }
  n168 = disable-structure shown="Disabled" {
    frame Disabled {
      n169 = local read "JS2_BTNS"() -> (w279:T5)
      n170 = local read "JS2_AXES"() -> (w278:T6)
      n171 = Unbundle By Name(w278) -> ("axis 1 (x)"=w277:dbl, "axis 2 (y)"=w276:dbl)
      n172 = Unbundle By Name(w279) -> ("Button 5"=w275:bool)
      n173 = case shown="True" w275 {
        tunnel: w277 -> [_ w284]
        tunnel: w276 -> [_ w283]
        frame False {
          w280 = 0.0
          n174 = call "Servo_Pan_Tilt.vi"("Tilt_Servo_Position"=w280, "Pan_Servo_Position"=w280, "Tilt_Servo_Name"="Tilt_Servo", "Pan_Servo_Name"="Pan_Servo") -> ()
        }
        frame True {
          n175 = call "Servo_Pan_Tilt.vi"("Tilt_Servo_Position"=w283, "Pan_Servo_Position"=w284, "Tilt_Servo_Name"="Tilt_Servo", "Pan_Servo_Name"="Pan_Servo") -> ()
        }
      }
    }
    frame Enabled {
    }
  }
  n176 = disable-structure shown="Enabled" {
    frame Enabled {
      # "L2 Arm Down"
      # "Could use Analog\nTrigger to make \nsure we're in bounds."
      # "L1 Arm Up"
      # "Pilot Control for Arm Mechanism"
      n177 = local read "JS1_BTNS"() -> (w298:T5)
      n178 = Unbundle By Name(w298) -> ("Button 5"=w290:bool, "Button 7"=w289:bool)
      n179 = Build Array(w290, w289) -> (w288:bool[])
      n180 = Boolean Array To Number(Boolean array=w288) -> (number=w287:u32)
      n181 = case shown="0, Default" w287 {
        tunnel: [w318 0.1 w320] -> w297
        frame 0, Default {
          n182 = local read "ARM_HOME"() -> (w318:dbl)
        }
        frame 1 {
          # "Set Arm To\nMid-Position\nSlightly Higher"
        }
        frame 2 {
          # "Set Arm Down"
          n183 = local read "ARM_REV_LIMIT"() -> (w320:dbl)
        }
      }
      n184 = call <vilib>:"WPI_AnalogChannelRefNum Registry Get.vi"("refnum name"="Feeder_Arm_Analog") -> ("AIDeviceRef"=w316:T20)  [unwired: 1 in, 9 out]
      n185 = call <vilib>:"WPI_AnalogChannelGetVoltage.vi"("AIDeviceRef"=w316) -> ("Voltage"=w313:dbl)  [unwired: 1 in, 9 out]
      n186 = Subtract(x=w313, y=2.5) -> (x-y=w294:dbl)
      n187 = Negate(x=w294) -> (-x=w295:dbl)
      n188 = Divide(x=w295, y=2.5) -> (x/y=w292:dbl)
      n189 = Greater?(x="ARM_FWD_LIMIT", y=w292) -> (0:w308:bool)
      n190 = Less?(x="ARM_REV_LIMIT", y=w292) -> (x < y?=w310:bool)
      n191 = call-poly <vilib>:"PID.vi"("output range"=cluster{"output low":dbl, "output high":dbl} {"output low"=-0.75, "output high"=0.5}, "PID gains"=T19 {"proportional gain (Kc)"=3.0, "integral time (Ti, min)"=0.0, "derivative time (Td, min)"=0.0}, "process variable"=w292, "setpoint"=w297) -> ("output"=w301:dbl)  [unwired: 2 in, 5 out]
      n192 = Select(t=1.0, s=w308, f=0.0) -> (s? t:f=w306:dbl)
      n193 = Select(t=-1.0, s=w310, f=0.0) -> (s? t:f=w307:dbl)
      n194 = In Range and Coerce(upper limit=w306, x=w301, lower limit=w307) -> (coerced(x)=w291:dbl)  [unwired: 1 out]
      n195 = call <vilib>:"WPI_MotorControlRefNum Registry Get.vi"("refnum name"="Ball_Grabber_Arm") -> ("MotorControlDevRef"=w317:T12)  [unwired: 1 in, 9 out]
      n196 = Negate(x=w291) -> (-x=w296:dbl)
      n197 = local write "Feeder_Arm_Speed"(w296) -> ()
      n198 = call <vilib>:"WPI_MotorControlSetOutput.vi"("Output"=w296, "MotorControlDevRef"=w317) -> ()  [unwired: 3 in, 7 out]
    }
    frame Disabled {
    }
  }
  n199 = disable-structure shown="Disabled" {
    frame Disabled {
      # "Victor Probably Dead!"
      # "Test w/ Arcade Driving First"
      # "Test w/ Arcade Driving First"
      # "Test w/ Arcade Driving First"
      n200 = local read "JS2_BTNS"() -> (w326:T5)
      n201 = Unbundle By Name(w326) -> ("Button 3"=w325:bool)
      n202 = local read "JS2_AXES"() -> (w338:T6)
      n203 = local read "JS2_BTNS"() -> (w337:T5)
      n204 = Unbundle By Name(w338) -> ("axis 2 (y)"=w322:dbl)
      n205 = case shown="True" w325 {
        tunnel: w322 -> [_ w342]
        tunnel: [0.0 w341] -> w328
        frame False {
        }
        frame True {
          n206 = local read "Drive_Reduce"() -> (w340:dbl)
          n207 = Divide(x=w342, y=w340) -> (x/y=w341:dbl)
        }
      }
      n208 = Unbundle By Name(w337) -> ("Button 4"=w336:bool)
      n209 = Negate(x=w322) -> (-x=w321:dbl)
      n210 = case shown="True" w336 {
        tunnel: w321 -> [_ w350]
        tunnel: [0.0 w349] -> w334
        frame False {
        }
        frame True {
          n211 = local read "Drive_Reduce"() -> (w348:dbl)
          n212 = Divide(x=w350, y=w348) -> (x/y=w349:dbl)
        }
      }
      n213 = call <vilib>:"WPI_MotorControlRefNum Registry Get.vi"("refnum name"="Shoot_Feeder") -> ("MotorControlDevRef"=w329:T12)  [unwired: 9 in, 1 out]
      n214 = call <vilib>:"WPI_MotorControlSetOutput.vi"("Output"=w328, "MotorControlDevRef"=w329) -> ()  [unwired: 7 in, 3 out]
      n215 = call <vilib>:"WPI_MotorControlRefNum Registry Get.vi"("refnum name"="Shooter") -> ("MotorControlDevRef"=w335:T12)  [unwired: 9 in, 1 out]
      n216 = local read "JS2_BTNS"() -> (w324:T5)
      n217 = Unbundle By Name(w324) -> ("Button 2"=w323:bool)
      n218 = call <vilib>:"WPI_MotorControlSetOutput.vi"("Output"=w334, "MotorControlDevRef"=w335) -> ()  [unwired: 7 in, 3 out]
      n219 = case shown="True" w323 {
        tunnel: w321 -> [_ w346]
        tunnel: [0.0 w345] -> w331
        frame False {
        }
        frame True {
          n220 = local read "Drive_Reduce"() -> (w344:dbl)
          n221 = Divide(x=w346, y=w344) -> (x/y=w345:dbl)
        }
      }
      n222 = call <vilib>:"WPI_MotorControlRefNum Registry Get.vi"("refnum name"="Ball_Sucker") -> ("MotorControlDevRef"=w332:T12)  [unwired: 9 in, 1 out]
      n223 = call <vilib>:"WPI_MotorControlSetOutput.vi"("Output"=w331, "MotorControlDevRef"=w332) -> ()  [unwired: 7 in, 3 out]
    }
    frame Enabled {
    }
  }
  n224 = disable-structure shown="Disabled" {
    frame Disabled {
      # "Test w/ Arcade Driving First"
      n225 = local read "JS2_BTNS"() -> (w353:T5)
      n226 = local read "JS2_AXES"() -> (w354:T6)
      n227 = Unbundle By Name(w353) -> ("Button 6"=w352:bool)
      n228 = Unbundle By Name(w354) -> ("axis 2 (y)"=w351:dbl)
      n229 = case shown="True" w352 {
        tunnel: w351 -> [_ w361]
        tunnel: [0.0 w360] -> w355
        frame False {
        }
        frame True {
          n230 = Divide(x=w361, y=1) -> (x/y=w360:dbl)
        }
      }
      n231 = call <vilib>:"WPI_MotorControlRefNum Registry Get.vi"("refnum name"="Ball_Grabber_Arm") -> ("MotorControlDevRef"=w357:T12)  [unwired: 9 in, 1 out]
      n232 = call <vilib>:"WPI_MotorControlSetOutput.vi"("Output"=w355, "MotorControlDevRef"=w357) -> ()  [unwired: 7 in, 3 out]
    }
    frame Enabled {
    }
  }
  n233 = disable-structure shown="Enabled" {
    frame Enabled {
      # "Co-Pilot Start/Select\nBattery Disengage for\nBalancing."
      n234 = local read "JS2_BTNS"() -> (w366:T5)
      n235 = Unbundle By Name(w366) -> ("Button 9"=w365:bool, "Button 10"=w364:bool)
      n236 = Build Array(w365, w364) -> (w363:bool[])
      n237 = Boolean Array To Number(Boolean array=w363) -> (number=w367:u32)
      n238 = case shown="3" w367 {
        tunnel: [WPI_RelayValue."Off" ("RelayValue") WPI_RelayValue."On" ("RelayValue")] -> w362
        frame 0, Default {
        }
        frame 3 {
        }
      }
      n239 = local read "Battery_Relay"() -> (w368:T1)
      n240 = call <vilib>:"WPI_RelaySet.vi"("RelayValue"=w362, "RelayDevRef"=w368) -> ()  [unwired: 8 in, 2 out]
    }
    frame Disabled {
    }
  }
  n241 = disable-structure shown="Disabled" {
    frame Disabled {
      # "Co-Pilot Reduced Belt Button Conrol"
      # "Pilot Reduced Belt Button Control"
      # "Master Control of Speeds"
      n242 = case shown="0, Default" {
        selector: _ -> [_ _ _ _ _ _ _ _ _]
        tunnel: [0 0.5 0.75 1 0.75 0.875 0.25 0.375 0.5] -> _
        frame 0, Default {
          # "Could keep shooter \nat -0.1"
        }
        frame 1 {
        }
        frame 2 {
        }
        frame 4 {
        }
        frame 5 {
          # "100+50/2"
        }
        frame 6 {
          # "72+100/2"
        }
        frame 8 {
        }
        frame 9 {
          # "50+25/2"
        }
        frame 10 {
          # "25+75/2"
        }
      }
      n243 = local read "JS2_BTNS"() -> (w382:T5)
      n244 = local read "JS1_BTNS"() -> (w371:T5)
      n245 = Unbundle By Name(w382) -> ("Button 1"=w377:bool, "Button 2"=w378:bool, "Button 3"=w379:bool, "Button 4"=w380:bool)
      n246 = Unbundle By Name(w371) -> ("Button 1"=w376:bool, "Button 2"=w375:bool, "Button 3"=w374:bool, "Button 4"=w373:bool)
      n247 = Build Array(w377, w378, w379, w380) -> (w381:bool[])
      n248 = Build Array(w376, w375, w374, w373) -> (w372:bool[])
      n249 = Boolean Array To Number(Boolean array=w381) -> (number=w385:u32)
      n250 = Boolean Array To Number(Boolean array=w372) -> (number=w384:u32)
      n251 = Greater Than 0?(x=w384) -> (x > 0?=w383:bool)
      n252 = case shown="False" w383 {
        tunnel: w384 -> [_ w400]
        tunnel: w385 -> [w399 _]
        tunnel: [w399 w400] -> _
        frame False {
        }
        frame True {
        }
      }
      n253 = disable-structure shown="Disabled" {
        disable-tunnel: [w398 _] -> _
        disable-tunnel: [w397 _] -> _
        disable-tunnel: [w393 _] -> _
        disable-tunnel: [w392 _] -> _
        disable-tunnel: [w389 _] -> _
        frame Disabled {
          w394 = -0.05
          w388 = 0.05
          # "Co-Pilot Feeder Control"
          # "Pilot Feeder Control"
          # "Pilot Has Feeder Master Control"
          n254 = local read "JS1_AXES"() -> (w387:T6)
          n255 = local read "JS2_AXES"() -> (w386:T6)
          n256 = Unbundle By Name(w387) -> ("axis 3 (throttle)"=w393:dbl, "axis 4"=w392:dbl)
          n257 = Unbundle By Name(w386) -> ("axis 3 (throttle)"=w398:dbl, "axis 4"=w397:dbl)
          n258 = In Range and Coerce(upper limit=w388, x=w392, lower limit=w394) -> (In Range?=w395:bool)  [unwired: 1 out]
          n259 = In Range and Coerce(upper limit=w388, x=w393, lower limit=w394) -> (In Range?=w396:bool)  [unwired: 1 out]
          n260 = Not(x=w395) -> (.not. x?=w390:bool)
          n261 = Not(x=w396) -> (.not. x?=w391:bool)
          n262 = Or(x=w391, y=w390) -> (x .or. y?=w389:bool)
        }
        frame Enabled {
        }
      }
    }
    frame Enabled {
    }
  }
